vi "ListColor.vi"() -> ()   [LabVIEW 2015]
panel:
  in  "Array":u8[](array[numeric])=[0, 102, 255]
  out "B":u8[](array[numeric])
  out "G":u8[](array[numeric])
  out "R":u8[](array[numeric])
  out "Color":u32[](array[colorbox])
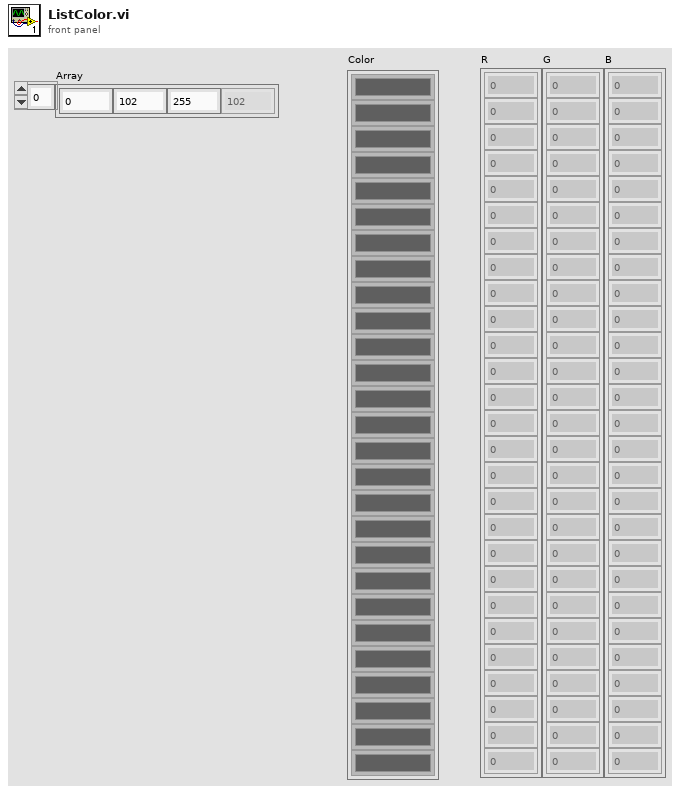
[diagram p1: front panel]
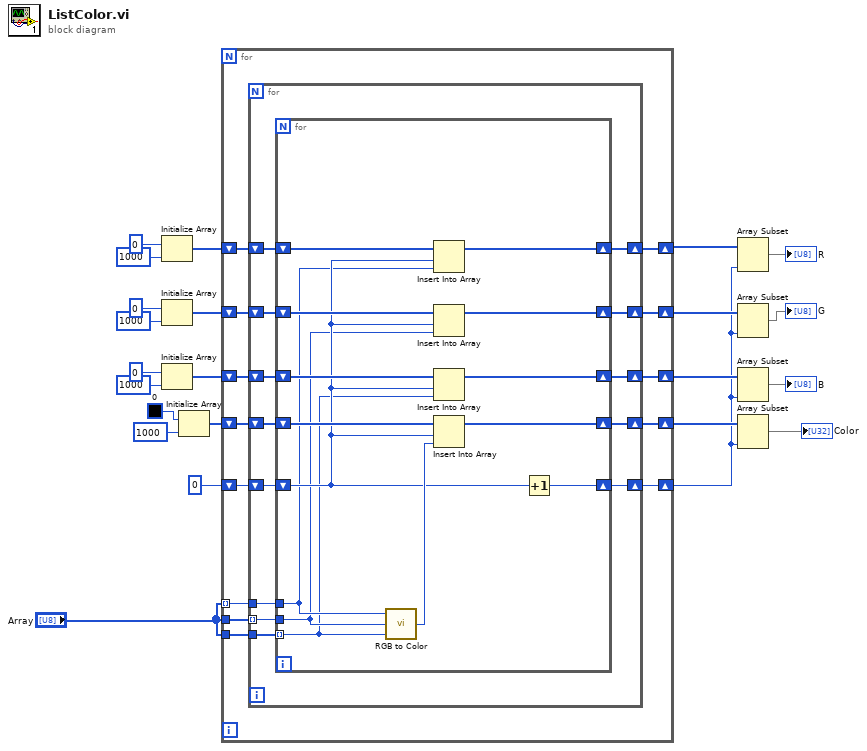
[diagram p0: block diagram]
diagram:
  n1 = Initialize Array(u8 0 ("R"), 1000 ("dimension size")) -> (w14:u8[])
  n2 = Initialize Array(u8 0 ("R"), 1000 ("dimension size")) -> (w9:u8[])
  n3 = Initialize Array(u8 0 ("R"), 1000 ("dimension size")) -> (w8:u8[])
  n4 = Initialize Array(u32 0 ("Array 2"), 1000 ("dimension size")) -> (w20:u32[])
  n5 = for {
    tunnel: "Array" -> [w36] mode=indexing
    tunnel: "Array" -> [w35]
    tunnel: "Array" -> [w34]
    shift-right: [w32] -> w1
    shift-left: 0 ("dimension size") -> [w31]
    shift-right: [w30] -> w18
    shift-left: w20 -> [w33]
    shift-right: [w26] -> w7
    shift-left: w14 -> [w29]
    shift-right: [w25] -> w3
    shift-left: w9 -> [w28]
    shift-right: [w24] -> w2
    shift-left: w8 -> [w27]
    n6 = for {
      tunnel: w36 -> [w49]
      tunnel: w35 -> [w48] mode=indexing
      tunnel: w34 -> [w47]
      shift-right: [w45] -> w32
      shift-left: w31 -> [w44]
      shift-right: [w43] -> w30
      shift-left: w33 -> [w46]
      shift-right: [w39] -> w26
      shift-left: w29 -> [w42]
      shift-right: [w38] -> w25
      shift-left: w28 -> [w41]
      shift-right: [w37] -> w24
      shift-left: w27 -> [w40]
      n7 = for {
        tunnel: w49 -> [w55]
        tunnel: w48 -> [w54]
        tunnel: w47 -> [w53] mode=indexing
        shift-right: [w62] -> w45
        shift-left: w44 -> [w56]
        shift-right: [w60] -> w43
        shift-left: w46 -> [w63]
        shift-right: [w50] -> w39
        shift-left: w42 -> [w59]
        shift-right: [w51] -> w38
        shift-left: w41 -> [w58]
        shift-right: [w52] -> w37
        shift-left: w40 -> [w57]
        n8 = call <vilib>:"RGB to Color.vi"("B"=w53, "G"=w54, "R"=w55) -> ("Color"=w61:u32)
        n9 = Insert Into Array(array=w59, index=w56, new element=w55) -> (w50:u8[])
        n10 = Insert Into Array(array=w58, index=w56, new element=w54) -> (w51:u8[])
        n11 = Insert Into Array(array=w57, index=w56, new element=w53) -> (w52:u8[])
        n12 = Insert Into Array(array=w63, index=w56, new element=w61) -> (w60:u32[])
        n13 = Increment(x=w56) -> (x+1=w62:i32)
      }
    }
  }
  n14 = Array Subset(array=w7, length=w1) -> (→"R":u8[])  [unwired: 1 in]
  n15 = Array Subset(array=w3, length=w1) -> (→"G":u8[])  [unwired: 1 in]
  n16 = Array Subset(array=w2, length=w1) -> (→"B":u8[])  [unwired: 1 in]
  n17 = Array Subset(array=w18, length=w1) -> (→"Color":u32[])  [unwired: 1 in]
